vi "convertUnitToRing.vi"(10 "Units":T1=enum."From TEDS") -> (2 "DAQmx units (Ring)":i32(ring)=10348 items=["Volts"=10348, "Amps"=10342, "Deg F"=10144, "Deg C"=10143, "Deg R"=10145, "Kelvins"=10325, "Strain"=10299, "Ohms"=10384, "Hz"=10373, "Seconds"=10364, "Meters"=10219, "Inches"=10379, "Degrees"=10146, "Radians"=10273, "Ticks"=10304, "g"=10186, "m/s^2"=12470, "m/s"=15959, "in/s"=15960, "Pascals"=10081, "Newtons"=15875, "Pounds"=15876, "kgf"=15877, "psi"=15879, "bar"=15880, "Nm"=15881, "oz-in"=15882, "lb-in"=15883, "lb-ft"=15884, "Volts/Volt"=15896, "mVolts/Volt"=15897, "From TEDS"=12516])   [LabVIEW 2013, in "DAQmx(AI).lvclass"]
uses:
  DAQmx(AI).lvclass
  Typedefs/Units -- Enum.ctl
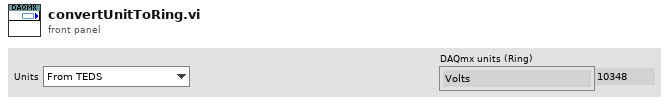
[diagram p1: front panel]
types:
  T1 = typedef "DAQmx(AI).lvclass/Units -- Enum.ctl" = enum16{"Volts", "Amps", "Deg F", "Deg C", "Deg R", "Kelvins", "Strain", "Ohms", "Hz", "Seconds", "Meters", "Inches", "Degrees", "Radians", "Ticks", "g", "m/s^2", "m/s", "in/s", "Pascals", "Newtons", "Pounds", "kgf", "psi", "bar", "Nm", "oz-in", "lb-in", "lb-ft", "Volts/Volt", "mVolts/Volt", "From TEDS"}
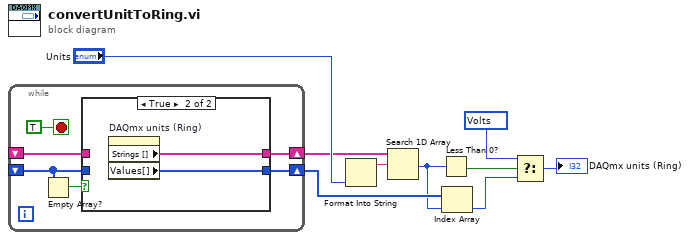
[diagram p0: block diagram]
diagram:
  w3 = 10348 items=["Volts"=10348, "Amps"=10342, "Deg F"=10144, "Deg C"=10143, "Deg R"=10145, "Kelvins"=10325, "Strain"=10299, "Ohms"=10384, "Hz"=10373, "Seconds"=10364, "Meters"=10219, "Inches"=10379, "Degrees"=10146, "Radians"=10273, "Ticks"=10304, "g"=10186, "m/s^2"=12470, "m/s"=15959, "in/s"=15960, "Pascals"=10081, "Newtons"=15875, "Pounds"=15876, "kgf"=15877, "psi"=15879, "bar"=15880, "Nm"=15881, "oz-in"=15882, "lb-in"=15883, "lb-ft"=15884, "Volts/Volt"=15896, "mVolts/Volt"=15897, "From TEDS"=12516] ("DAQmx units (Ring)")
  n1 = while {
    shift-right: [w14] -> w6
    shift-left: _ -> [w11]
    shift-right: [w15] -> w8
    shift-left: _ -> [w10]
    stop <- TRUE stop-if-true
    n2 = Empty Array?(array=w11) -> (empty?=w12:bool)
    n3 = case shown="True" w12 {
      tunnel: [w17 w19] -> w15
      tunnel: [w16 w18] -> w14
      tunnel: w11 -> [w16 _]
      tunnel: w10 -> [w17 _]
      frame False {
      }
      frame True {
        n4 = property on="DAQmx units (Ring)" class="Ring (strict)"() -> ("Strings []"=w19:string[], "Values[]"=w18:i32[])  [unwired: 2 in, 2 out]
      }
    }
  }
  n5 = Format Into String("Units") -> (resulting string=w7:string)  [unwired: 3 in, 1 out]
  n6 = Search 1D Array(1D array=w8, element=w7) -> (index of element=w5:i32)  [unwired: 1 in]
  n7 = Less Than 0?(x=w5) -> (x < 0?=w4:bool)
  n8 = Index Array(array=w6, index=w5) -> (element=w2:i32)
  n9 = Select(t=w3, s=w4, f=w2) -> (s? t:f=→"DAQmx units (Ring)":i32)
